vi "referenceModel.vi"(8 "path":cluster{"x":dbl, "y":dbl}[](array[cluster]), 11 "e_b":dbl[](array[numeric])) -> (2 "eta_r":dbl[](array[numeric]))   [LabVIEW 2014]
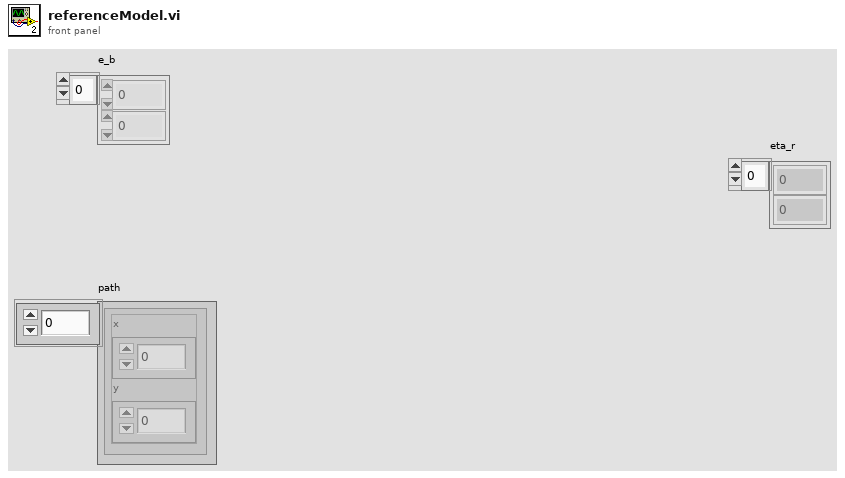
[diagram p1: front panel]
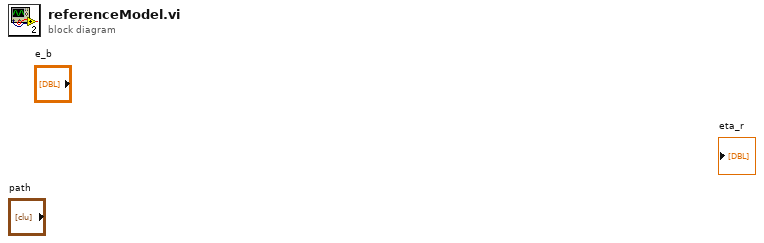
[diagram p0: block diagram]
diagram:
